vi "IO_MFA_StepDir_Read_PulseCount1.vi"() -> (3 "PulseCounter Init":i32)   [LabVIEW 2018]
panel:
  out "error PulseCounter Init":errorcluster
  out "AAABuild":i32
  in  "MintController":refnum<k7>(container)
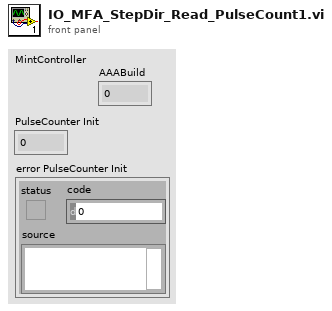
[diagram p1: front panel]
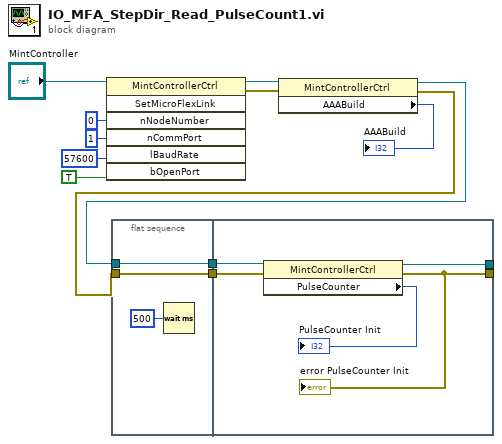
[diagram p0: block diagram]
diagram:
  n1 = invoke class="MintControllerCtrl" method="SetMicroFlexLink"(reference="MintController", "nNodeNumber"=i16 0, "nCommPort"=i16 1, "lBaudRate"=57600, "bOpenPort"=TRUE) -> (reference out=w12:refnum<k7>, error out=w6:errorcluster)  [unwired: 2 in, 5 out]
  n2 = flat-sequence {
    tunnel: [w15] -> w4
    tunnel: w3 -> [w15]
    tunnel: w2 -> [w13]
    tunnel: [w13] -> w1
    tunnel: w4 -> [w20]
    tunnel: [w17] -> _
    tunnel: [w16] -> _
    tunnel: w1 -> [w19]
    frame #0 {
      n3 = Wait (ms)(milliseconds to wait=u32 500) -> ()  [unwired: 1 out]
    }
    frame #1 {
      n4 = property class="MintControllerCtrl"(reference=w19, error in=w20) -> (reference out=w16:refnum<k7>, error out=w17:errorcluster, "PulseCounter"=→"PulseCounter Init":i32)
      "error PulseCounter Init" <- w17
    }
  }
  n5 = property class="MintControllerCtrl"(reference=w12, error in=w6) -> (reference out=w2:refnum<k7>, error out=w3:errorcluster, "AAABuild"=→"AAABuild":i32)
